vi "FTW-Client-Ask.vi"(0 "FTW-Client In":refnum<class "FTW-Client.lvclass">, 5 "Header":string, 7 "Body":string, 9 "Timeout":i32=1000 format="%dmsec", 11 "error in":errorcluster) -> (4 "FTW-Client Out":refnum<class "FTW-Client.lvclass">, 6 "Response Header":string, 8 "Response Body":string, 10 "Timed out?":bool, 14 "Roundtrip Time":dbl format="%.6fsec", 15 "error out":errorcluster)   [LabVIEW 2013, in "FTW-Client.lvclass"]
uses:
  FTW-Client.lvclass
  FTW-Client.lvclass/FTW-Client.ctl
  Endpoint/FTW-Endpoint.lvclass
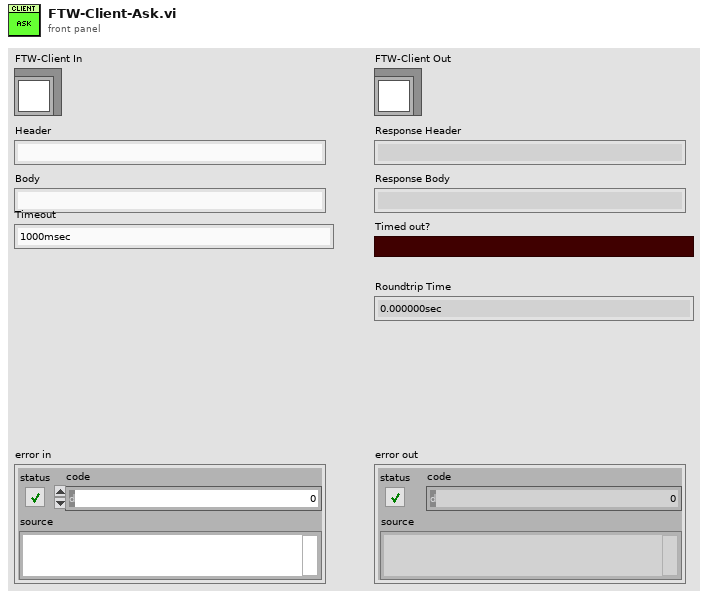
[diagram p1: front panel]
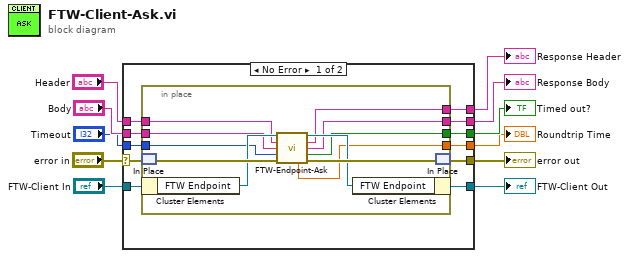
[diagram p0: block diagram]
diagram:
  n1 = case shown="No Error" "error in" {
    selector: "error in" -> [w20 w35]
    tunnel: [w19 w35] -> w8
    tunnel: [w21 w34] -> w10
    tunnel: "FTW-Client In" -> [w22 w34]
    tunnel: "Header" -> [w18 _]
    tunnel: [w15 _] -> w1
    tunnel: "Body" -> [w17 _]
    tunnel: [w14 _] -> w2
    tunnel: "Timeout" -> [w16 _]
    tunnel: [w13 _] -> w4
    tunnel: [w12 _] -> w3
    frame No Error {
      n2 = in-place {
        in-place-border: w18 -> [w29]
        in-place-border: w17 -> [w28]
        in-place-border: w16 -> [w27]
        in-place-border: [w25] -> w15
        in-place-border: [w26] -> w14
        in-place-border: [w24] -> w13
        in-place-border: [w23] -> w12
        n3 = in-place-match #1(w20) -> (w33:errorcluster)
        n4 = in-place-cluster #2(w22) -> ("FTW Endpoint"=w31:refnum<class "FTW-Endpoint.lvclass">)
        n5 = call-dynamic "FTW-Endpoint-Ask.vi"("FTW Endpoint"=w31, "Request Header"=w29, "Request Body"=w28, "Timeout"=w27, "error in"=w33) -> ("FTW Endpoint out"=w30:refnum<class "FTW-Endpoint.lvclass">, "Response Header"=w26:string, "Response Body"=w25:string, "Timed out?"=w24:bool, "Roundtrip Time"=w23:dbl, "error out"=w32:errorcluster)  [unwired: 5 in]
        n6 = in-place-cluster #2("FTW Endpoint"=w30) -> (w21:refnum<class "FTW-Client.lvclass">)
        n7 = in-place-match #1(w32) -> (w19:errorcluster)
      }
    }
    frame Error {
    }
  }
  "FTW-Client Out" <- w10
  "error out" <- w8
  "Response Header" <- w2
  "Response Body" <- w1
  "Timed out?" <- w4
  "Roundtrip Time" <- w3
